vi "重复执行.vi"(8 "error in":errorcluster caption="错误输入") -> (0 "error out":errorcluster caption="错误输出")   [LabVIEW 2016]
uses:
  <vilib>/Utility/config.llb/Write Key (Boolean).vi
  <vilib>/Utility/config.llb/NI_LVConfig.lvlib
  kernel32.dll
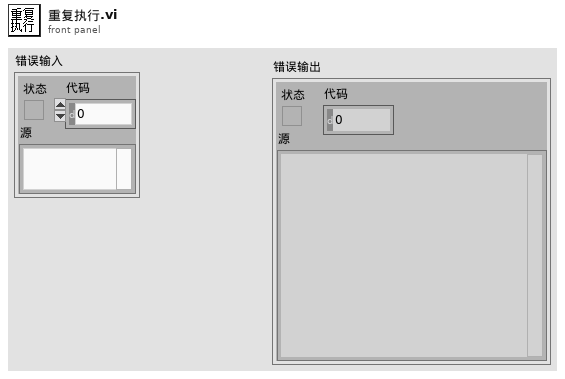
[diagram p1: front panel]
types:
  T1 = typedef "NI_LVConfig.lvlib/Config Data RefNum.ctl" = refnum<k1>
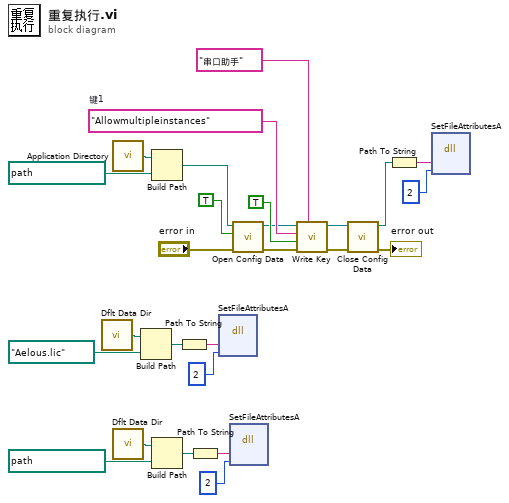
[diagram p0: block diagram]
diagram:
  w26 = "Allowmultipleinstances"  # 键1
  n1 = call <vilib>:"Dflt Data Dir.vi"() -> ("App:Default Data Directory"=w8:path)
  n2 = call <vilib>:"Application Directory.vi"() -> ("Application Directory"=w23:path)
  n3 = call <vilib>:"Dflt Data Dir.vi"() -> ("App:Default Data Directory"=w4:path)
  n4 = Build Path(base path=w8, name or relative path=path "Aelous.lic" ("default name")) -> (appended path=w6:path)
  n5 = Build Path(base path=w23, name or relative path=path "串口助手.ini" ("default name")) -> (appended path=w12:path)
  n6 = Build Path(base path=w4, name or relative path=path "串口助手.ini" ("default name")) -> (appended path=w5:path)
  n7 = Path To String(path=w6) -> (string=w9:string)
  n8 = Path To String(path=w5) -> (string=w3:string)
  n9 = dll-call lib="kernel32.dll" fn="SetFileAttributesA"("Filename"=w9, "FileAttributes"=2) -> ()  [unwired: 6 in, 2 out]
  n10 = dll-call lib="kernel32.dll" fn="SetFileAttributesA"("Filename"=w3, "FileAttributes"=2) -> ()  [unwired: 6 in, 2 out]
  n11 = call <vilib>:"Open Config Data.vi"("error in (no error)"="error in", "create file if necessary (T)"=TRUE, "configuration file path"=w12) -> ("error out"=w21:errorcluster, "refnum"=w22:T1)  [unwired: 7 out]
  n12 = call-poly <vilib>:"Write Key.vi"("section"="串口助手", "error in (no error)"=w21, "value"=TRUE, "key"=w26, "refnum"=w22) -> ("error out"=w19:errorcluster, "refnum out"=w20:T1)  [unwired: 1 in, 4 out]
  n13 = call <vilib>:"Close Config Data.vi"("error in (no error)"=w19, "refnum"=w20) -> ("error out"=→"error out":errorcluster, "file path"=w16:path)  [unwired: 1 in, 7 out]
  n14 = Path To String(path=w16) -> (string=w17:string)
  n15 = dll-call lib="kernel32.dll" fn="SetFileAttributesA"("Filename"=w17, "FileAttributes"=2) -> ()  [unwired: 6 in, 2 out]
